vi "RunPythonStateDet.vi"(8 "error in (no error)":errorcluster, 10 "filepath":string, 11 "Compiler Settings":T1={"Python Path"=path "", "Main File"="mainscript.py", "Meta File"="metascript.txt", "Aux File"="auxscript.py", "Pre File"="metascript.txt"}) -> (0 "error out":errorcluster, 2 "standard error":string, 3 "standard output":string)   [LabVIEW 2019]
uses:
  PulseCompiler/CompilerSettings.ctl
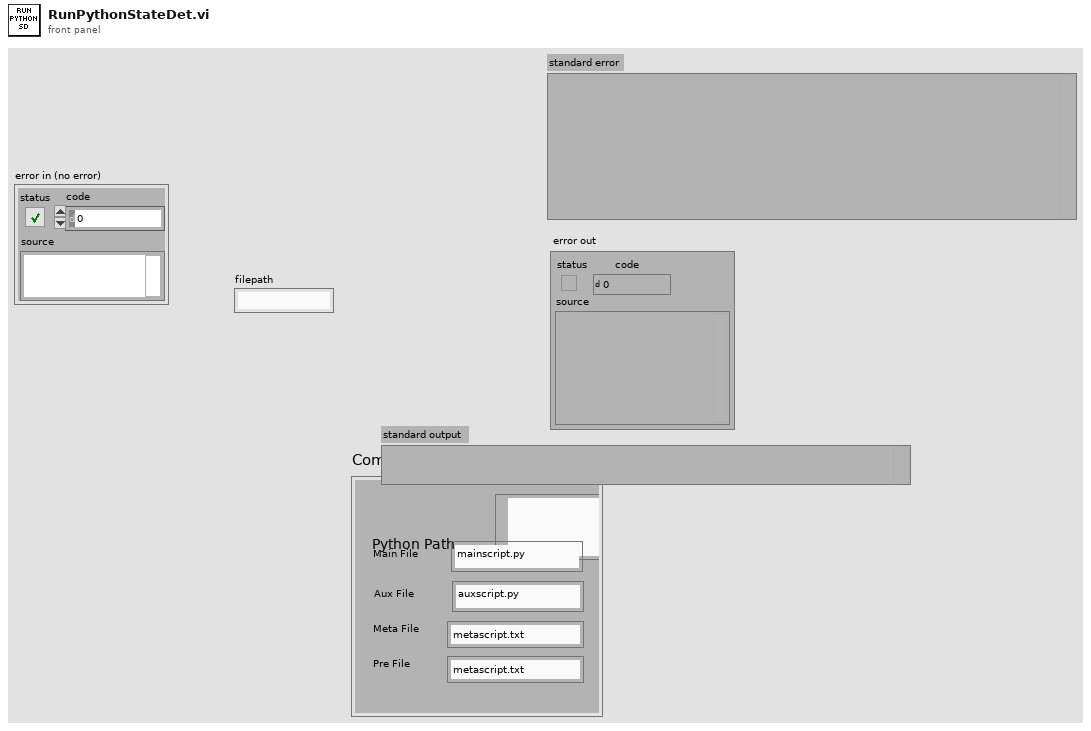
[diagram p1: front panel]
types:
  T1 = typedef "CompilerSettings.ctl" = cluster{"Python Path":path, "Main File":string, "Meta File":string, "Aux File":string, "Pre File":string}
  T2 = cluster{"filepath":string, "update":bool, "genimage":bool}
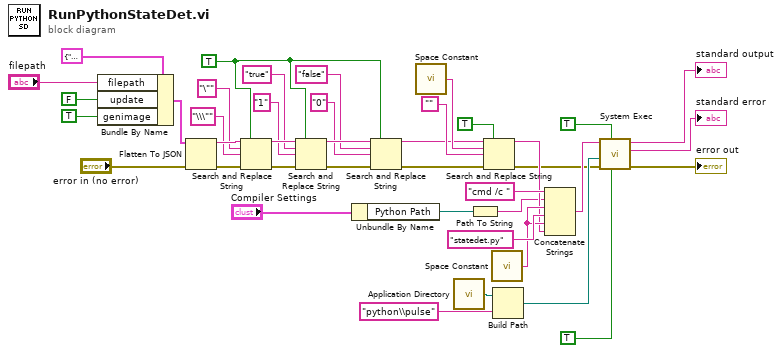
[diagram p0: block diagram]
diagram:
  w9 = TRUE ("replace all? (F)")
  n1 = Bundle By Name(cluster=T2 {"filepath"="", "update"=TRUE, "genimage"=TRUE}, "filepath"="filepath", "update"=FALSE, "genimage"=TRUE) -> (w17:T2)
  n2 = Flatten To JSON(anything=w17, error in (no error)="error in (no error)") -> (JSON string=w27:string, 11:w26:errorcluster)  [unwired: 1 in]
  n3 = Search and Replace String(replace all?=w9, input string=w27, search string="\"", replace string="\\\"" ("replace string (\"\")"), error in=w26) -> (result string=w14:string, error out=w11:errorcluster)  [unwired: 3 in, 2 out]
  n4 = Search and Replace String(replace all?=w9, input string=w14, search string="true", replace string="1" ("replace string (\"\")"), error in=w11) -> (result string=w10:string, error out=w6:errorcluster)  [unwired: 3 in, 2 out]
  n5 = Unbundle By Name("Compiler Settings") -> ("Python Path"=w16:path)
  n6 = Search and Replace String(replace all?=w9, input string=w10, search string="false", replace string="0" ("replace string (\"\")"), error in=w6) -> (result string=w4:string, error out=w5:errorcluster)  [unwired: 3 in, 2 out]
  n7 = call <vilib>:"Space Constant.vi"() -> ("String"=w23:string)
  n8 = call <vilib>:"Application Directory.vi"() -> ("Application Directory"=w31:path)
  n9 = Path To String(path=w16) -> (string=w15:string)
  n10 = Search and Replace String(replace all?=TRUE ("replace all? (F)"), input string=w4, search string=w23, replace string="", error in=w5) -> (result string=w21:string, error out=w20:errorcluster)  [unwired: 3 in, 2 out]
  n11 = call <vilib>:"Space Constant.vi"() -> ("String"=w28:string)
  n12 = Build Path(base path=w31, name or relative path="python\\pulse") -> (appended path=w33:path)
  n13 = Concatenate Strings("cmd /c " ("string"), w15, w28, "statedet.py" ("name or relative path"), w28, w21) -> (w30:string)
  n14 = call <vilib>:"System Exec.vi"("run minimized? (F)"=TRUE, "wait until completion? (T)"=TRUE, "error in (no error)"=w20, "working directory"=w33, "command line"=w30) -> ("error out"=→"error out":errorcluster, "standard error"=→"standard error":string, "standard output"=→"standard output":string)  [unwired: 3 in, 1 out]
